vi "Begin.vi"() -> (0 "Error Out":errorcluster)   [LabVIEW 2019]
doc: "This VI creates the roboRIO file tree (if necessary), opens device references, sets constants, clears hardware sticky faults, defines static VI references, and resets gobal variables."
uses:
  <vilib>/Rock Robotics/WPI/DriverStation/WPI_DriverStationRobotMode2.ctl
  dsdata.vi
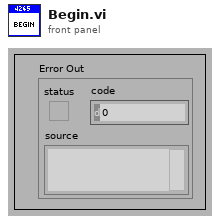
[diagram p1: front panel]
types:
  T1 = typedef "WPI_DriverStationRobotMode2.ctl" = enum16{"Autonomous Disabled", "Autonomous Enabled", "Teleop Disabled", "Teleop Enabled", "Disconnected", "Finish", "Test Disabled", "Test Enabled", "Emergency Stopped"}
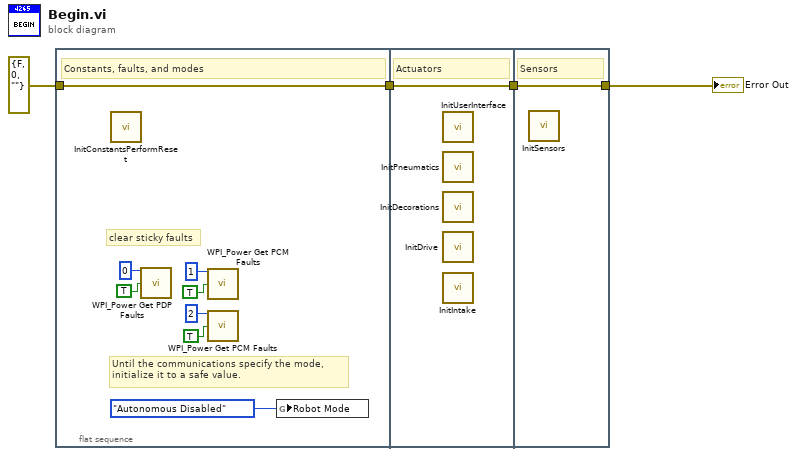
[diagram p0: block diagram]
diagram:
  n1 = flat-sequence {
    tunnel: [w12] -> w4
    tunnel: errorcluster {"status"=FALSE, "code"=0, "source"=""} ("error in") -> [w12]
    tunnel: w4 -> [w13]
    tunnel: [w13] -> w2
    tunnel: w2 -> [w14]
    tunnel: [w14] -> w1
    frame #0 {
      # "clear sticky faults"
      # "Until the communications specify the mode,\ninitialize it to a safe value."
      # "Constants, faults, and modes"
      n2 = call "InitConstantsPerformReset.vi"() -> ()  [unwired: 12 in]
      n3 = call <vilib>:"WPI_Power Get PDP Faults.vi"("Power Distribution Panel (0)"=u8 0, "Clear Sticky Faults"=TRUE) -> ()  [unwired: 9 in, 5 out]
      n4 = call <vilib>:"WPI_Power Get PCM Faults.vi"("Pneumatics Control Module (0)"=u8 1, "Clear Sticky Faults"=TRUE) -> ()  [unwired: 10 in, 4 out]
      n5 = call <vilib>:"WPI_Power Get PCM Faults.vi"("Pneumatics Control Module (0)"=u8 2, "Clear Sticky Faults"=TRUE) -> ()  [unwired: 10 in, 4 out]
      n6 = global write "dsdata.vi" "Robot Mode"(WPI_DriverStationRobotMode2."Autonomous Disabled" ("Robot Mode")) -> ()
    }
    frame #1 {
      # "Actuators"
      n7 = call "InitUserInterface.vi"() -> ()  [unwired: 12 in]
      n8 = call "InitPneumatics.vi"() -> ()  [unwired: 12 in]
      n9 = call "InitDecorations.vi"() -> ()  [unwired: 12 in]
      n10 = call "InitDrive.vi"() -> ()  [unwired: 1 in]
      n11 = call "InitIntake.vi"() -> ()  [unwired: 1 in]
    }
    frame #2 {
      # "Sensors"
      n12 = call "InitSensors.vi"() -> ()  [unwired: 1 in]
    }
  }
  "Error Out" <- w1
